vi "Calculate Counter And Protections Main.vi"(6 "timeout ms":i32, 7 "Frame Count":i32, 8 "error in (no error)":errorcluster, 9 "Signals":T9, 10 "Protections":T1, 11 "Frames in":T2[](array[typedef]) {"Protection Configurations"."CRC Channels"."Data Type" items=["Signed", "Unsigned", "IEEE Float"]}) -> (0 "error out":errorcluster, 1 "Tick Count(uSec)":u32, 2 "Frames":T10[](array[typedef]) {"payload" format="%x"; "timestamp" format="%<%.7X\n%x>T"; "type" items=["CAN Data"=0, "CAN Remote"=1, "CAN Bus Error"=2, "CAN 2.0 Data"=8, "CAN FD Data"=16, "CAN FD+BRS Data"=24, "J1939 Data"=192, "Delay"=224, "Log Trigger"=225, "Start Trigger"=226]; "identifier" format="%x"}, 3 "Frames out":T2[](array[typedef]) {"Protection Configurations"."CRC Channels"."Data Type" items=["Signed", "Unsigned", "IEEE Float"]})   [LabVIEW 2015, in "Protection and Counter Support Engine.lvlib"]
uses:
  Protection and Counter Support Engine.lvlib
  <vilib>/xnet/xnet.llb/XNET Frame CAN.ctl
  <vilib>/xnet/xnet.llb/XNET Frame Type CAN.ctl
  Types/RT Frame Settings.ctl
  Shared/Types/Exported Frame Type.ctl
  Types/RT Protection Configuration.ctl
  Shared/Types/Protection Type.ctl
  Shared/Types/XNET Signal Configuration.ctl
  Shared/Types/Exported Counter Settings.ctl
  Shared/Types/Exported Event Trigger Type.ctl
  <vilib>/NI/NIVS Inline Async API/_Data Access Engine/Data Access Engine/Types/Read.DVR.ctl
  <vilib>/NI/NIVS Inline Async API/_Data Access Engine/Access Type Classes/Read/Read.lvclass
  <vilib>/NI/NIVS Inline Async API/_Data Access Engine/Data Access Engine/Types/Write.DVR.ctl
  <vilib>/NI/NIVS Inline Async API/_Data Access Engine/Access Type Classes/Write/Write.lvclass
  <vilib>/NI/NIVS Inline Async API/_Data Access Engine/Access Type Classes/Read/Read.lvclass/Read.ctl
  <vilib>/NI/NIVS Inline Async API/_Data Access Engine/Access Type Classes/Write/Write.lvclass/Write.ctl
  <vilib>/NI/NIVS Inline Async API/_Data Access Engine/Data Access Engine/Methods/Write.Data.Buffer.vi
  <vilib>/NI/NIVS Inline Async API/_Data Access Engine/Data Access Engine/Methods/Write.Data.Commit.vi
  <vilib>/NI/NIVS Inline Async API/_Data Access Engine/Data Access Engine/Methods/Read.Data.Detect.vi
  <vilib>/NI/NIVS Inline Async API/_Data Access Engine/Access Type Classes/Write/Write.Buffer.vi
  <vilib>/NI/NIVS Inline Async API/_Data Access Engine/Access Type Classes/Write/Write.Commit.vi
  <vilib>/NI/NIVS Inline Async API/_Data Access Engine/Access Type Classes/Read/Read.ProcessData.Detect.vi
  <vilib>/xnet/xnet.llb/XNET Convert (Signal to Frame CAN).vi
  <vilib>/xnet/xnet.llb/XNET Convert (Signal to Frame Raw).vi
  <vilib>/NI/NIVS Inline Async API/_Data Access Engine/Data Access Engine/Data Access Engine.lvclass
  <vilib>/NI/NIVS Inline Async API/_Data Access Engine/Data Access Engine/Methods/Read.Data.vi
  Shared/Protection and Counter Support Shared.lvlib
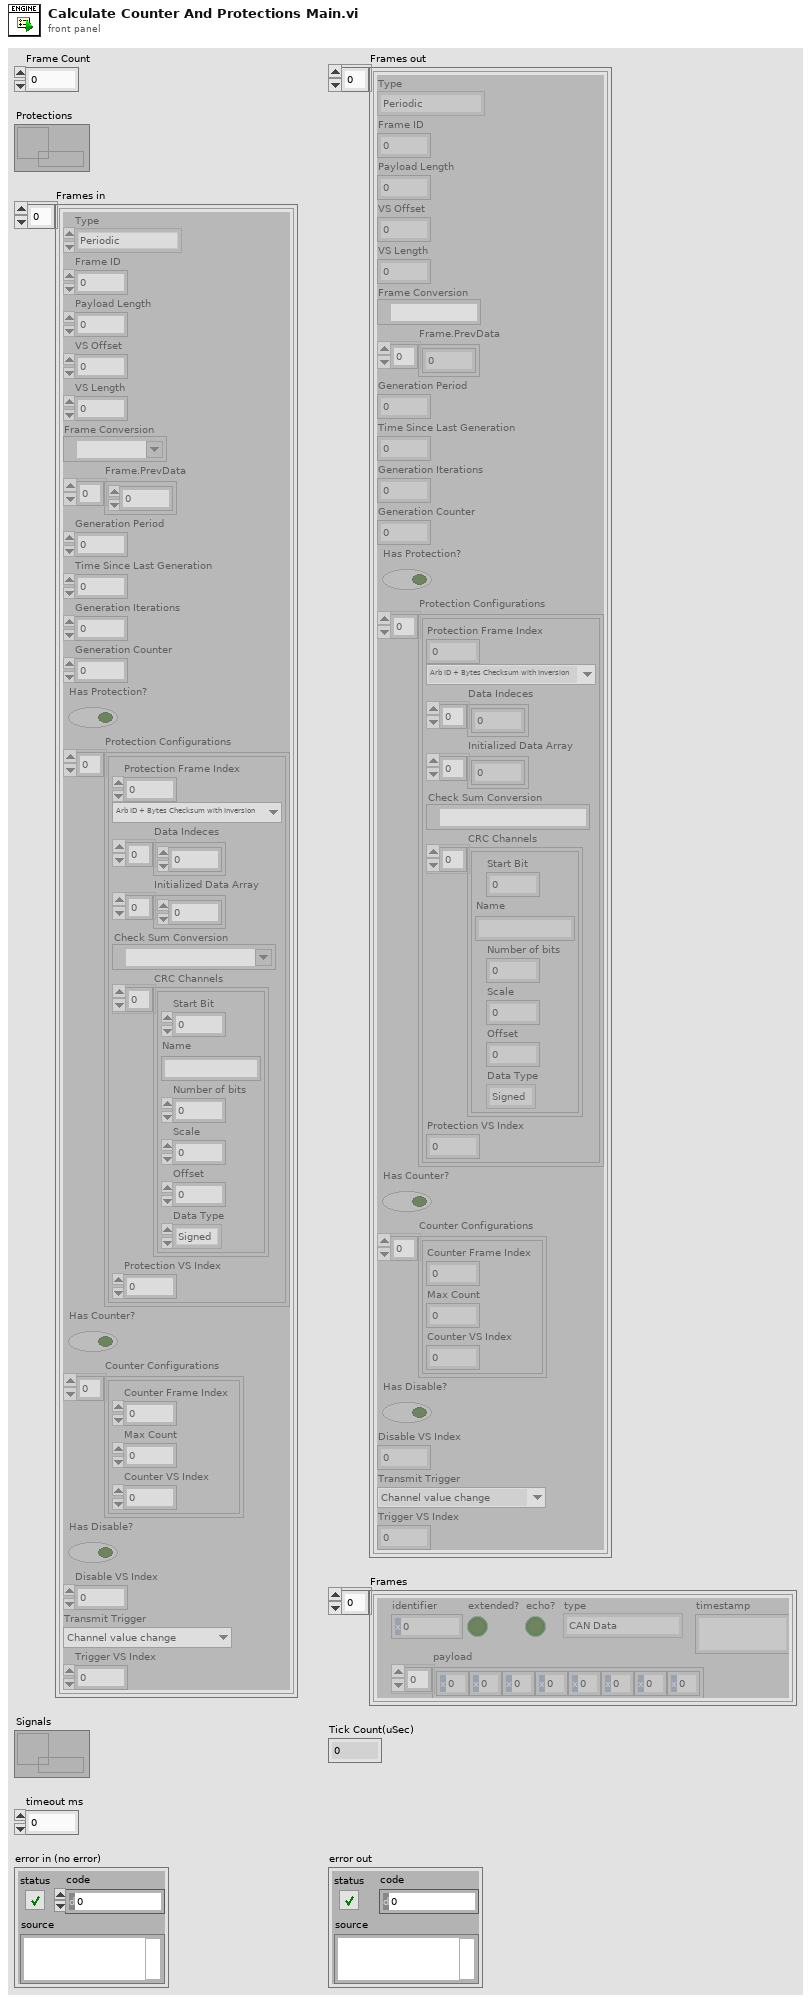
[diagram p1: front panel]
types:
  T1 = typedef "Data Access Engine.lvlib/Data Access Engine.lvclass/Write.DVR.ctl" = refnum<data-value>
  T2 = typedef "Protection and Counter Support Engine.lvlib/RT Frame Settings.ctl" = cluster{"Type":T3, "Frame ID":u32, "Payload Length":u32, "VS Offset":i32, "VS Length":i32, "Frame Conversion":refnum<k21>, "Frame.PrevData":dbl[], "Generation Period":u32, "Time Since Last Generation":u32, "Generation Iterations":u32, "Generation Counter":u32, "Has Protection?":bool, "Protection Configurations":T4[], "Has Counter?":bool, "Counter Configurations":T7[], "Has Disable?":bool, "Disable VS Index":i32, "Transmit Trigger":T8, "Trigger VS Index":i32}
  T3 = typedef "Protection and Counter Support Shared.lvlib/Exported Frame Type.ctl" = enum16{"Periodic", "Event", "Periodic/Event"}
  T4 = typedef "Protection and Counter Support Engine.lvlib/RT Protection Configuration.ctl" = cluster{"Protection Frame Index":i32, "Protection Type":T5, "Data Indeces":i32[], "Initialized Data Array":dbl[], "Check Sum Conversion":refnum<k21>, "CRC Channels":T6[], "Protection VS Index":i32}
  T5 = typedef "Protection and Counter Support Shared.lvlib/Protection Type.ctl" = enum16{"Arb ID + Bytes Checksum with Inversion", "Arb ID + Bytes CRC with Inversion", "Reversed Raw Signal Checksum with Inversion"}
  T6 = typedef "Protection and Counter Support Shared.lvlib/XNET Signal Configuration.ctl" = cluster{"Start Bit":i32, "Name":string, "Number of bits":i32, "Scale":dbl, "Offset":dbl, "Data Type":u32}
  T7 = typedef "Protection and Counter Support Shared.lvlib/Exported Counter Settings.ctl" = cluster{"Counter Frame Index":i32, "Max Count":dbl, "Counter VS Index":i32}
  T8 = typedef "Protection and Counter Support Shared.lvlib/Exported Event Trigger Type.ctl" = enum16{"Channel value change", "Trigger channel (not zero)", "Channel value change or trigger channel (not zero)", "Trigger channel (any value change)", "Channel value change or trigger channel (any value change)"}
  T9 = typedef "Data Access Engine.lvlib/Data Access Engine.lvclass/Read.DVR.ctl" = refnum<data-value>
  T10 = typedef "XNET Frame CAN.ctl" = cluster{"timestamp":timestamp, "payload":u8[], "identifier":u32, "type":T11, "extended?":bool, "echo?":bool}
  T11 = typedef "XNET Frame Type CAN.ctl" = u8
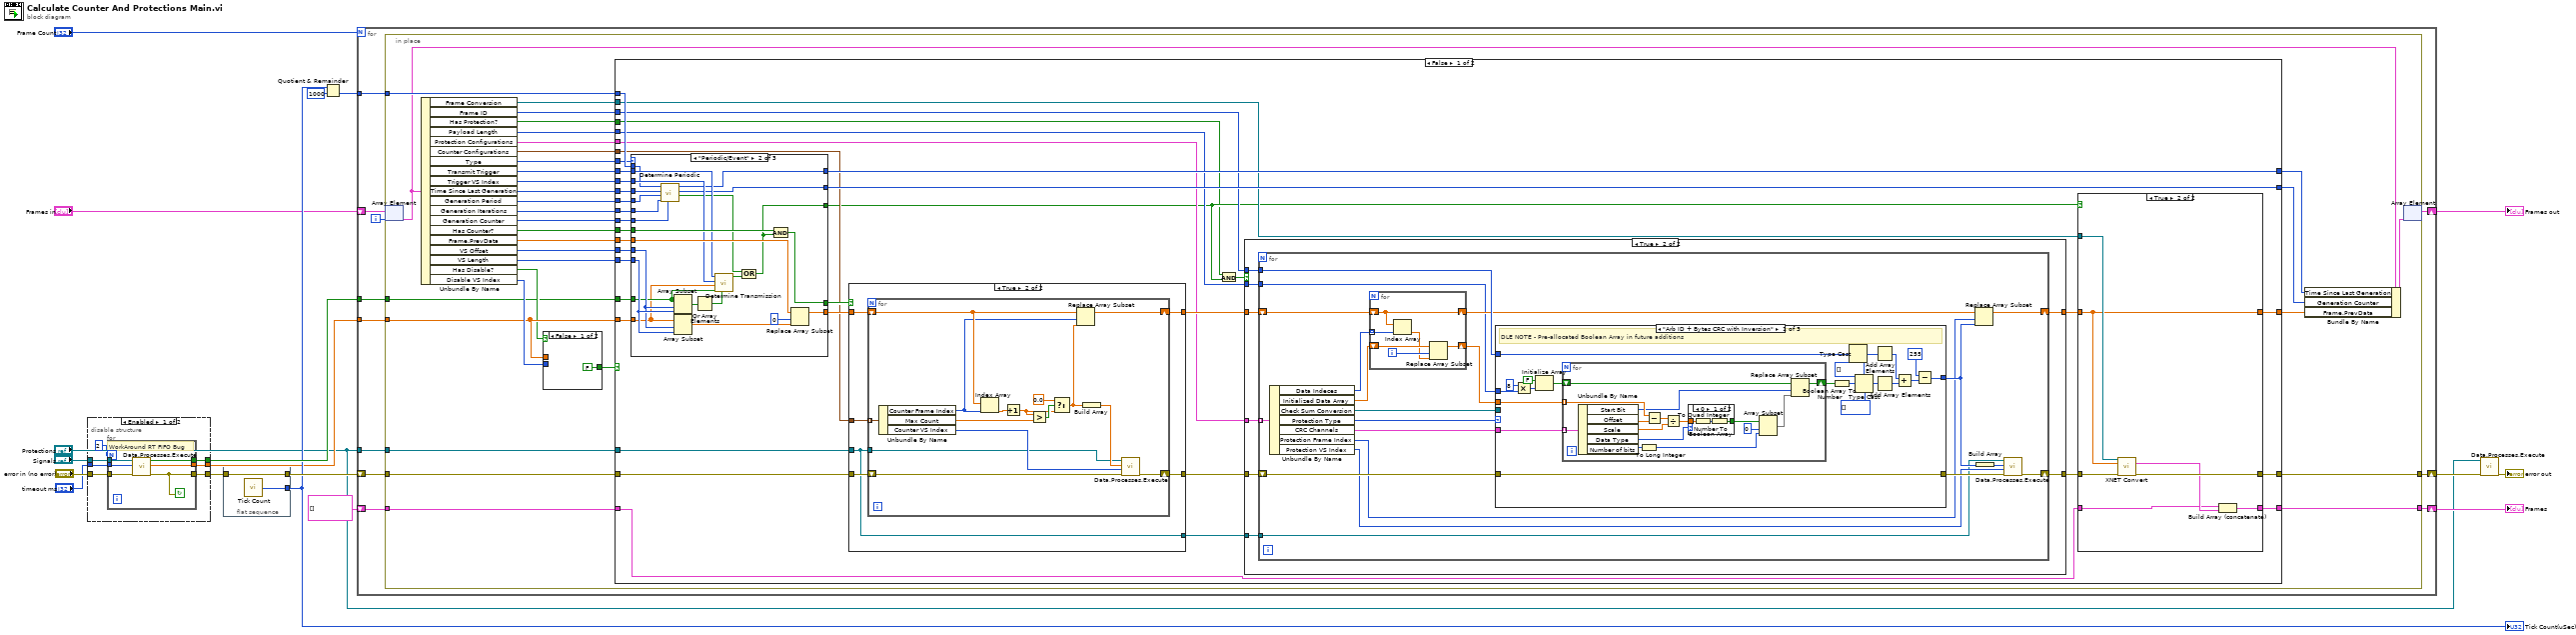
[diagram p0: block diagram]
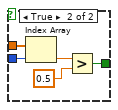
[diagram p2: hidden frame]
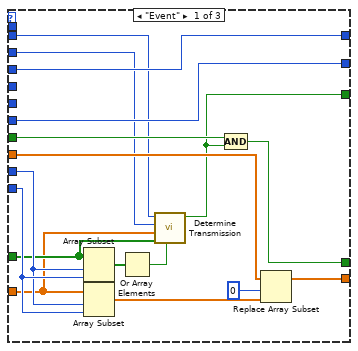
[diagram p3: hidden frame]
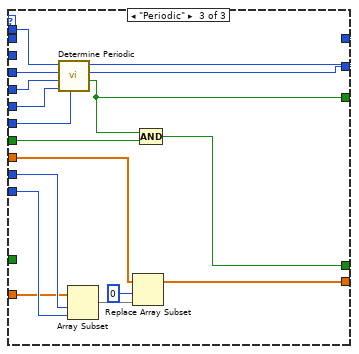
[diagram p4: hidden frame]
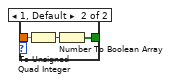
[diagram p7: hidden frame]
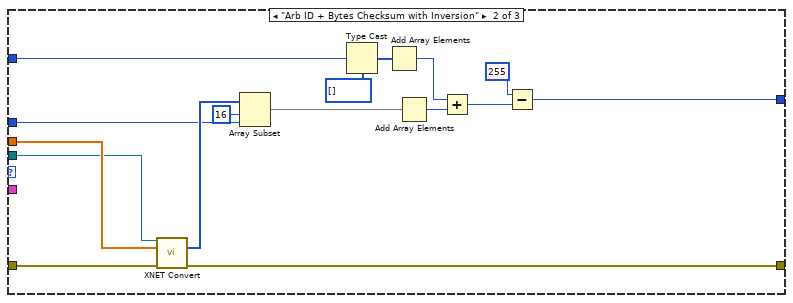
[diagram p8: hidden frame]
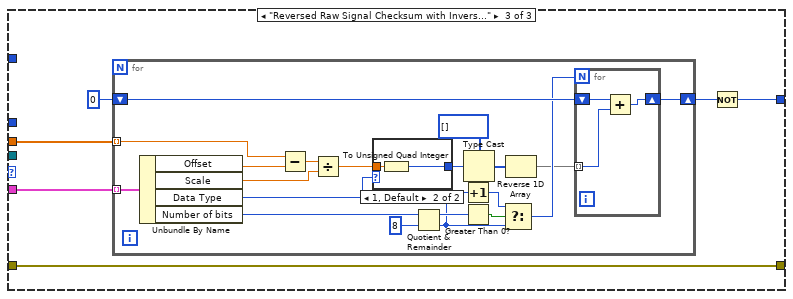
[diagram p9: hidden frame]
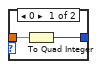
[diagram p10: hidden frame]
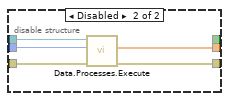
[diagram p13: hidden frame]
diagram:
  n1 = disable-structure shown="Enabled" {
    disable-tunnel: "timeout ms" -> [w25 w36]
    disable-tunnel: [w24 w35] -> w17
    disable-tunnel: [w23 w34] -> w3
    disable-tunnel: "error in (no error)" -> [w22 w33]
    disable-tunnel: "Signals" -> [w21 w32]
    disable-tunnel: [w19 _] -> w9
    frame Enabled {
      n2 = for {
        N: 2 -> [_]
        tunnel: w25 -> [w31]
        tunnel: [w30] -> w23
        tunnel: w21 -> [w28]
        tunnel: w22 -> [w29]
        tunnel: [w27] -> w24
        tunnel: [w26] -> w19
        stop <- w27 continue-if-true
        # "WorkAround RT FIFO Bug"
        n3 = call-poly <vilib>:"Data.Processes.Execute.vi"("error in (no error)"=w29, "timeout ms"=w31, "Ref"=w28) -> ("error out"=w27:errorcluster, "Values"=w30:dbl[], "Detect?"=w26:bool[])  [unwired: 5 in, 1 out]
      }
    }
    frame Disabled {
      n4 = call-poly <vilib>:"Data.Processes.Execute.vi"("error in (no error)"=w33, "timeout ms"=w36, "Ref"=w32) -> ("error out"=w35:errorcluster, "Values"=w34:dbl[])  [unwired: 6 in, 1 out]
    }
  }
  n5 = flat-sequence {
    tunnel: [w38] -> w8
    tunnel: [w37] -> w18
    tunnel: w17 -> [w37]
    frame #0 {
      n6 = call "Tick Count"() -> ("Tick Count(uSec)"=w38:u32)
    }
  }
  n7 = Quotient & Remainder(x=w8, y=u32 1000) -> (floor(x/y)=w11:u32)  [unwired: 1 out]
  n8 = for {
    N: "Frame Count" -> [_]
    tunnel: w3 -> [w46]
    shift-right: [w48] -> w15
    shift-left: w18 -> [w49]
    tunnel: w11 -> [w47]
    tunnel: "Protections" -> [w45]
    shift-right: [w42] -> w10
    shift-left: "Frames in" -> [w44]
    tunnel: w9 -> [w41]
    shift-right: [w40] -> w14
    shift-left: T10[] [] -> [w39]
    i -> [w43]
    n9 = in-place {
      in-place-border: w49 -> [w82]
      in-place-border: [w81] -> w48
      in-place-border: w47 -> [w77]
      in-place-border: w46 -> [w75]
      in-place-border: w45 -> [w70]
      in-place-border: w41 -> [w58]
      in-place-border: [w51] -> w40
      in-place-border: w39 -> [w50]
      n10 = in-place-array #1(w44, w43) -> (w63:T2)
      n11 = Unbundle By Name(w63) -> ("Frame Conversion"=w53:refnum<k21>, "Frame ID"=w54:u32, "Has Protection?"=w55:bool, "Payload Length"=w56:u32, "Protection Configurations"=w52:T4[], "Counter Configurations"=w57:T7[], "Type"=w61:T3, "Transmit Trigger"=w60:T8, "Trigger VS Index"=w59:i32, "Time Since Last Generation"=w71:u32, "Generation Period"=w72:u32, "Generation Iterations"=w66:u32, "Generation Counter"=w65:u32, "Has Counter?"=w78:bool, "Frame.PrevData"=w69:dbl[], "VS Offset"=w80:i32, "VS Length"=w79:i32, "Has Disable?"=w74:bool, "Disable VS Index"=w76:i32)
      n12 = case shown="False" w74 {
        tunnel: w76 -> [_ w88]
        tunnel: w75 -> [_ w87]
        tunnel: [FALSE w85] -> w73
        frame False {
        }
        frame True {
          n13 = Index Array(array=w87, index=w88) -> (element=w86:dbl)
          n14 = Greater?(x=w86, y=0.5 ("x")) -> (0:w85:bool)
        }
      }
      n15 = case shown="False" w73 {
        tunnel: w82 -> [w118 w348]
        tunnel: [w124 w348] -> w81
        tunnel: w80 -> [w102 _]
        tunnel: w79 -> [w103 _]
        tunnel: w78 -> [w123 _]
        tunnel: w77 -> [w110 _]
        tunnel: w72 -> [w120 _]
        tunnel: w75 -> [w100 _]
        tunnel: w71 -> [w111 w347]
        tunnel: w70 -> [w116 _]
        tunnel: w69 -> [w114 w345]
        tunnel: [w112 w345] -> w68
        tunnel: [w109 w347] -> w67
        tunnel: w66 -> [w107 _]
        tunnel: w65 -> [w108 w346]
        tunnel: [w106 w346] -> w64
        tunnel: w61 -> [w99 _]
        tunnel: w60 -> [w105 _]
        tunnel: w59 -> [w104 _]
        tunnel: w58 -> [w101 _]
        tunnel: w57 -> [w98 _]
        tunnel: w56 -> [w97 _]
        tunnel: w55 -> [w92 _]
        tunnel: w54 -> [w96 _]
        tunnel: w52 -> [w95 _]
        tunnel: w53 -> [w94 _]
        tunnel: [w90 w344] -> w51
        tunnel: w50 -> [w89 w344]
        frame False {
          n16 = case shown="\"Periodic/Event\"" w99 {
            tunnel: w123 -> [w142 w166 w183]
            tunnel: w120 -> [_ w150 w182]
            tunnel: [w141 w165 w181] -> w119
            tunnel: w114 -> [w140 w164 w180]
            tunnel: [w137 w161 w177] -> w113
            tunnel: w111 -> [w136 w149 w176]
            tunnel: w110 -> [_ w148 w175]
            tunnel: [w136 w147 w174] -> w109
            tunnel: w108 -> [w135 w152 w167]
            tunnel: w107 -> [_ w151 w168]
            tunnel: [w128 w143 w173] -> w93
            tunnel: [w135 w146 w172] -> w106
            tunnel: w105 -> [w130 w156 _]
            tunnel: w104 -> [w131 w157 _]
            tunnel: w103 -> [w134 w160 w171]
            tunnel: w102 -> [w133 w159 w170]
            tunnel: w101 -> [w127 w154 _]
            tunnel: w100 -> [w126 w153 w169]
            frame "Event" {
              n17 = Array Subset(array=w127, index=w133, length=w134) -> (w132:bool[])
              n18 = Array Subset(array=w126, index=w133, length=w134) -> (w138:dbl[])
              n19 = Or Array Elements(Boolean array=w132) -> (logical OR=w129:bool)
              n20 = call "Determine Transmission.vi"("Channel Value Change"=w129, "Detect?"=w127, "Values"=w126, "Trigger VS Index"=w131, "Transmit Trigger"=w130) -> ("Transmit"=w128:bool)  [unwired: 6 in]
              n21 = Compound Arithmetic op=AND(w142, w128) -> (w141:bool)
              n22 = Replace Array Subset(array=w140, new element=w138, index=0) -> (w137:dbl[])
            }
            frame "Periodic/Event" {
              n23 = call "Determine Periodic.vi"("Generation Counter"=w152, "Generation Iterations"=w151, "Generation Period"=w150, "Time Since Last Generation in"=w149, "Current Time"=w148) -> ("Tranmit"=w145:bool, "Generation Counter out"=w146:u32, "Time Since Last Generation out"=w147:u32)  [unwired: 4 in]
              n24 = Array Subset(array=w154, index=w159, length=w160) -> (w158:bool[])
              n25 = Array Subset(array=w153, index=w159, length=w160) -> (w162:dbl[])
              n26 = Or Array Elements(Boolean array=w158) -> (logical OR=w155:bool)
              n27 = call "Determine Transmission.vi"("Channel Value Change"=w155, "Detect?"=w154, "Values"=w153, "Trigger VS Index"=w157, "Transmit Trigger"=w156) -> ("Transmit"=w144:bool)  [unwired: 6 in]
              n28 = Compound Arithmetic op=OR(w145, w144) -> (w143:bool)
              n29 = Compound Arithmetic op=AND(w166, w143) -> (w165:bool)
              n30 = Replace Array Subset(array=w164, new element=w162, index=0) -> (w161:dbl[])
            }
            frame "Periodic" {
              n31 = call "Determine Periodic.vi"("Generation Counter"=w167, "Generation Iterations"=w168, "Generation Period"=w182, "Time Since Last Generation in"=w176, "Current Time"=w175) -> ("Tranmit"=w173:bool, "Generation Counter out"=w172:u32, "Time Since Last Generation out"=w174:u32)  [unwired: 4 in]
              n32 = Array Subset(array=w169, index=w170, length=w171) -> (w178:dbl[])
              n33 = Replace Array Subset(array=w180, new element=w178, index=0) -> (w177:dbl[])
              n34 = Compound Arithmetic op=AND(w173, w183) -> (w181:bool)
            }
          }
          n35 = case shown="True" w119 {
            tunnel: w113 -> [w186 w192]
            tunnel: [w186 w191] -> w122
            tunnel: w98 -> [_ w190]
            tunnel: w118 -> [w185 w189]
            tunnel: [w185 w188] -> w117
            tunnel: w116 -> [w184 w187]
            tunnel: [w184 w187] -> w115
            frame False {
            }
            frame True {
              n36 = for {
                shift-right: [w205] -> w191
                shift-left: w192 -> [w207]
                tunnel: w190 -> [w204] mode=indexing
                shift-right: [w194] -> w188
                shift-left: w189 -> [w195]
                tunnel: w187 -> [w193]
                n37 = Unbundle By Name(w204) -> ("Counter Frame Index"=w200:i32, "Max Count"=w206:dbl, "Counter VS Index"=w198:i32)
                n38 = Index Array(array=w207, index=w200) -> (element=w201:dbl)
                n39 = Increment(x=w201) -> (x+1=w199:dbl)
                n40 = Greater?(x=w199, y=w206) -> (0:w203:bool)
                n41 = Select(t=0.0, s=w203, f=w199) -> (s? t:f=w197:dbl)
                n42 = Replace Array Subset(array=w207, new element=w197, index=w200) -> (w205:dbl[])
                n43 = Build Array(w197) -> (w196:dbl[])
                n44 = call-poly <vilib>:"Data.Processes.Execute.vi"("error in (no error)"=w195, "Offset"=w198, "Values"=w196, "Ref"=w193) -> ("error out"=w194:errorcluster)  [unwired: 7 in]
              }
            }
          }
          n45 = Compound Arithmetic op=AND(w92, w93) -> (w91:bool)
          n46 = case shown="True" w91 {
            tunnel: w96 -> [_ w217]
            tunnel: w117 -> [w209 w216]
            tunnel: [w209 w215] -> w125
            tunnel: w122 -> [w208 w214]
            tunnel: w95 -> [_ w213]
            tunnel: [w208 w212] -> w121
            tunnel: w115 -> [_ w211]
            tunnel: w97 -> [_ w210]
            frame False {
            }
            frame True {
              n47 = for {
                tunnel: w217 -> [w237]
                tunnel: w213 -> [w234] mode=indexing
                shift-right: [w226] -> w215
                shift-left: w216 -> [w236]
                shift-right: [w235] -> w212
                shift-left: w214 -> [w231]
                tunnel: w211 -> [w219]
                tunnel: w210 -> [w218]
                n48 = Unbundle By Name(w234) -> ("Data Indeces"=w232:i32[], "Initialized Data Array"=w229:dbl[], "Check Sum Conversion"=w221:refnum<k21>, "Protection Type"=w222:T5, "CRC Channels"=w233:T6[], "Protection Frame Index"=w220:i32, "Protection VS Index"=w223:i32)
                n49 = for {
                  shift-right: [w242] -> w230
                  shift-left: w231 -> [w242]
                  tunnel: w232 -> [w243] mode=indexing
                  shift-right: [w238] -> w228
                  shift-left: w229 -> [w241]
                  i -> [w240]
                  n50 = Index Array(array=w242, index=w243) -> (element=w239:dbl)
                  n51 = Replace Array Subset(array=w241, new element=w239, index=w240) -> (w238:dbl[])
                }
                n52 = case shown="\"Arb ID + Bytes CRC with Inversion\"" w222 {
                  tunnel: w237 -> [w261 w298 _]
                  tunnel: [w256 w293 w302] -> w225
                  tunnel: w236 -> [w252 w292 w301]
                  tunnel: [w252 w291 w301] -> w227
                  tunnel: w233 -> [w250 _ w304]
                  tunnel: w228 -> [w251 w288 w303]
                  tunnel: w221 -> [_ w287 _]
                  tunnel: w218 -> [w246 w286 _]
                  frame "Arb ID + Bytes CRC with Inversion" {
                    # "DLE NOTE - Pre-allocated Boolean Array in future additions"
                    n53 = Multiply(x=u32 8, y=w246) -> (x*y=w247:u32)
                    n54 = Initialize Array(FALSE, w247) -> (w249:bool[])
                    n55 = for {
                      tunnel: w250 -> [w278] mode=indexing
                      shift-right: [w269] -> w255
                      shift-left: w249 -> [w271]
                      tunnel: w251 -> [w268] mode=indexing
                      n56 = Unbundle By Name(w278) -> ("Start Bit"=w265:i32, "Offset"=w277:dbl, "Scale"=w275:dbl, "Data Type"=w267:u32, "Number of bits"=w273:i32)
                      n57 = To Long Integer(number=w273) -> (32bit integer=w264:i32)
                      n58 = Subtract(x=w268, y=w277) -> (x-y=w276:dbl)
                      n59 = Divide(x=w276, y=w275) -> (x/y=w274:dbl)
                      n60 = case shown="0" w267 {
                        tunnel: w274 -> [w281 w284]
                        tunnel: [w279 w282] -> w266
                        frame 0 {
                          n61 = To Quad Integer(1:w281) -> (0:w280:i64)
                          n62 = Number To Boolean Array(number=w280) -> (Boolean array=w279:bool[])
                        }
                        frame 1, Default {
                          n63 = To Unsigned Quad Integer(1:w284) -> (0:w283:u64)
                          n64 = Number To Boolean Array(number=w283) -> (Boolean array=w282:bool[])
                        }
                      }
                      n65 = Array Subset(array=w266, index=0, length=w264) -> (w270:bool[])
                      n66 = Replace Array Subset(array=w271, new element=w270, index=w265) -> (w269:bool[])
                    }
                    n67 = Boolean Array To Number(Boolean array=w255) -> (number=w254:u64)
                    n68 = Type Cast(type=u8[] [], x=w261) -> (*(type *) &x=w260:u8[])
                    n69 = Type Cast(type=u8[] [], x=w254) -> (*(type *) &x=w244:u8[])
                    n70 = Add Array Elements(numeric array=w260) -> (sum=w259:u8)
                    n71 = Add Array Elements(numeric array=w244) -> (sum=w263:u8)
                    n72 = Add(x=w259, y=w263) -> (x+y=w258:u8)
                    n73 = Subtract(x=u8 255, y=w258) -> (x-y=w256:u8)
                  }
                  frame "Arb ID + Bytes Checksum with Inversion" {
                    n74 = call-poly <vilib>:"XNET Convert.vi"("session in"=w287, "signal data"=w288, "error in (no error)"=w292) -> ("frame data"=w289:u8[], "error out"=w291:errorcluster)  [unwired: 10 in, 1 out]
                    n75 = Array Subset(array=w289, index=16 ("length"), length=w286) -> (w285:u8[])
                    n76 = Type Cast(type=u8[] [], x=w298) -> (*(type *) &x=w297:u8[])
                    n77 = Add Array Elements(numeric array=w297) -> (sum=w296:u8)
                    n78 = Add Array Elements(numeric array=w285) -> (sum=w300:u8)
                    n79 = Add(x=w296, y=w300) -> (x+y=w295:u8)
                    n80 = Subtract(x=u8 255, y=w295) -> (x-y=w293:u8)
                  }
                  frame "Reversed Raw Signal Checksum with Inversion" {
                    n81 = for {
                      tunnel: w304 -> [w326] mode=indexing
                      tunnel: w303 -> [w323] mode=indexing
                      shift-right: [w320] -> w305
                      shift-left: u8 0 -> [w321]
                      n82 = Unbundle By Name(w326) -> ("Offset"=w325:dbl, "Scale"=w324:dbl, "Data Type"=w322:u32, "Number of bits"=w318:i32)
                      n83 = Subtract(x=w323, y=w325) -> (x-y=w317:dbl)
                      n84 = Divide(x=w317, y=w324) -> (x/y=w316:dbl)
                      n85 = case shown="1, Default" w322 {
                        tunnel: w316 -> [w331 w333]
                        tunnel: [w330 w332] -> w319
                        frame 0 {
                          n86 = To Quad Integer(1:w331) -> (0:w330:i64)
                        }
                        frame 1, Default {
                          n87 = To Unsigned Quad Integer(1:w333) -> (0:w332:u64)
                        }
                      }
                      n88 = Quotient & Remainder(x=w318, y=8) -> (x-y*floor(x/y)=w313:i32, floor(x/y)=w311:i32)
                      n89 = Increment(x=w311) -> (x+1=w312:i32)
                      n90 = Greater Than 0?(x=w313) -> (x > 0?=w314:bool)
                      n91 = Type Cast(type=u8[] [], x=w319) -> (*(type *) &x=w308:u8[])
                      n92 = Select(t=w312, s=w314, f=w311) -> (s? t:f=w310:i32)
                      n93 = Reverse 1D Array(array=w308) -> (reversed array=w307:u8[])
                      n94 = for {
                        N: w310 -> [_]
                        tunnel: w307 -> [w328] mode=indexing
                        shift-right: [w327] -> w320
                        shift-left: w321 -> [w329]
                        n95 = Add(x=w329, y=w328) -> (x+y=w327:u8)
                      }
                    }
                    n96 = Not(x=w305) -> (.not. x?=w302:u8)
                  }
                }
                n97 = Replace Array Subset(array=w230, new element=w225, index=w220) -> (w235:dbl[])
                n98 = Build Array(w225) -> (w224:u8[])
                n99 = call-poly <vilib>:"Data.Processes.Execute.vi"("error in (no error)"=w227, "Offset"=w223, "Values"=w224, "Ref"=w219) -> ("error out"=w226:errorcluster)  [unwired: 7 in]
              }
            }
          }
          n100 = case shown="True" w93 {
            tunnel: w125 -> [w336 w343]
            tunnel: [w336 w340] -> w124
            tunnel: w121 -> [w335 w341]
            tunnel: w94 -> [_ w342]
            tunnel: [w335 w341] -> w112
            tunnel: [w334 w338] -> w90
            tunnel: w89 -> [w334 w337]
            frame False {
            }
            frame True {
              n101 = call-poly <vilib>:"XNET Convert.vi"("session in"=w342, "signal data"=w341, "error in (no error)"=w343) -> ("frame data"=w339:T10[], "error out"=w340:errorcluster)  [unwired: 9 in, 2 out]
              n102 = Build Array (concatenate)(w337, w339) -> (w338:T10[])
            }
          }
        }
        frame True {
        }
      }
      n103 = Bundle By Name(cluster=w63, "Time Since Last Generation"=w67, "Generation Counter"=w64, "Frame.PrevData"=w68) -> (w62:T2)
      n104 = in-place-array #1(w62) -> (w42:T2[])  [unwired: 1 out]
    }
  }
  "Frames" <- w14
  "Frames out" <- w10
  n105 = call-poly <vilib>:"Data.Processes.Execute.vi"("error in (no error)"=w15, "Ref"="Protections") -> ("error out"=→"error out":errorcluster)  [unwired: 9 in]
  "Tick Count(uSec)" <- w8
